vi "Timer.vi"(8 "error in":errorcluster, 10 "limit":dbl, 11 "timer state":T1) -> (0 "error out":errorcluster, 2 "limit reached":bool, 3 "elapsed":dbl)   [LabVIEW 2015]
doc: "Count time in seconds.\nStart- start counting.\nStop- reset timer and stop counting."
uses:
  Controls/timer status.ctl
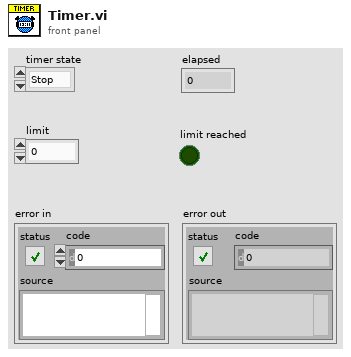
[diagram p1: front panel]
types:
  T1 = typedef "timer status.ctl" = enum16{"Stop", "Start"}
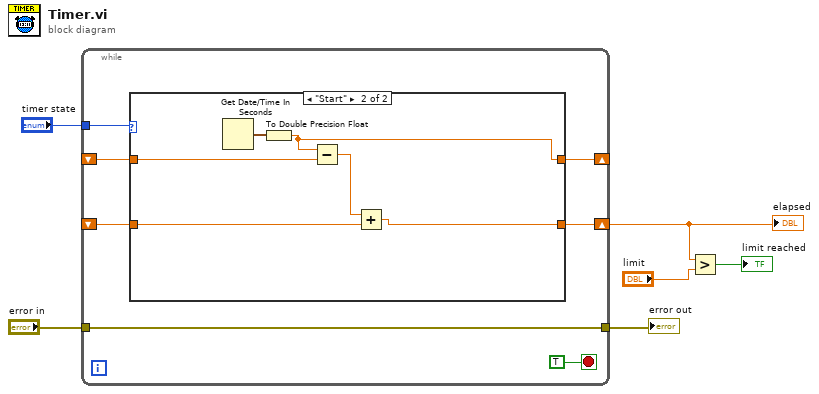
[diagram p0: block diagram]
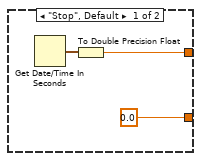
[diagram p2: hidden frame]
diagram:
  n1 = while {
    tunnel: "timer state" -> [w13]
    shift-right: [w12] -> _
    shift-left: _ -> [w10]
    shift-right: [w11] -> w5
    shift-left: _ -> [w9]
    tunnel: "error in" -> [w7]
    tunnel: [w7] -> w1
    stop <- TRUE stop-if-true
    n2 = case shown="\"Start\"" w13 {
      tunnel: [w15 w17] -> w12
      tunnel: [0.0 w18] -> w11
      tunnel: w10 -> [_ w21]
      tunnel: w9 -> [_ w19]
      frame "Stop", Default {
        n3 = Get Date/Time In Seconds() -> (seconds since 1Jan1904=w16:timestamp)
        n4 = To Double Precision Float(number=w16) -> (double precision float=w15:dbl)
      }
      frame "Start" {
        n5 = Get Date/Time In Seconds() -> (seconds since 1Jan1904=w22:timestamp)
        n6 = To Double Precision Float(number=w22) -> (double precision float=w17:dbl)
        n7 = Subtract(x=w17, y=w21) -> (x-y=w20:dbl)
        n8 = Add(x=w20, y=w19) -> (x+y=w18:dbl)
      }
    }
  }
  "elapsed" <- w5
  "error out" <- w1
  n9 = Greater?(x=w5, y="limit") -> (0:→"limit reached":bool)
